vi "Send Message.vi"   [LabVIEW 2015, in "NI_AWS_SQS.lvlib" / "Queue.lvclass"]
uses:
  Queue.lvclass
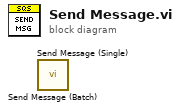
[diagram p0: block diagram]
diagram:
  n1 = call "Send Message (Batch).vi"() -> ()  [unwired: 8 in, 4 out]
  n2 = call "Send Message (Single).vi"() -> ()  [unwired: 8 in, 4 out]
